vi "Filter Targets.vi"(6 "Camera Type":enum16{"206", "1011"}(ring), 9 "Targets":T2[](array[typedef]), 10 "Score Limits":T3, 11 "Image Size":cluster{i32, i32}) -> (3 "Filtered Targets":T1[](array[typedef]))   [LabVIEW 2011]
uses:
  Target Data.ctl
  Target.ctl
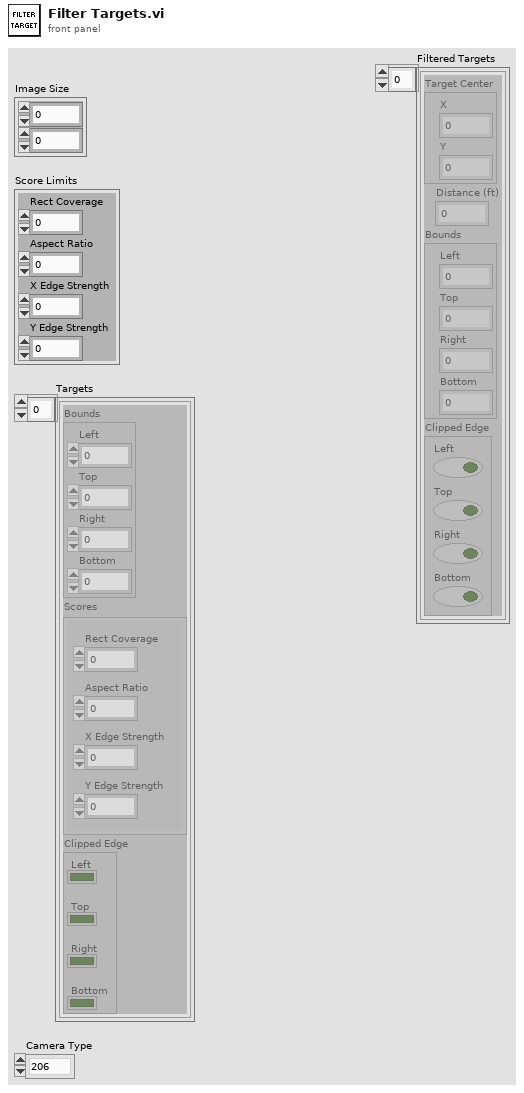
[diagram p1: front panel]
types:
  T1 = typedef "Target.ctl" = cluster{"Target Center":cluster{"X":dbl, "Y":dbl}, "Distance (ft)":dbl, "Bounds":cluster{"Left":dbl, "Top":dbl, "Right":dbl, "Bottom":dbl}, "Clipped Edge":cluster{"Left":bool, "Top":bool, "Right":bool, "Bottom":bool}}
  T2 = typedef "Target Data.ctl" = cluster{"Bounds":cluster{"Left":dbl, "Top":dbl, "Right":dbl, "Bottom":dbl}, "Scores":cluster{"Rect Coverage":dbl, "Aspect Ratio":dbl, "X Edge Strength":dbl, "Y Edge Strength":dbl}, "Clipped Edge":cluster{"Left":bool, "Top":bool, "Right":bool, "Bottom":bool}}
  T3 = cluster{"Rect Coverage":dbl, "Aspect Ratio":dbl, "X Edge Strength":dbl, "Y Edge Strength":dbl}
  T4 = cluster{"Left":dbl, "Top":dbl, "Right":dbl, "Bottom":dbl}
  T5 = cluster{"Left":bool, "Top":bool, "Right":bool, "Bottom":bool}
  T6 = cluster{"Target Center":cluster{"X":dbl, "Y":dbl}, "Distance (ft)":dbl, "Bounds":cluster{"Left":dbl, "Top":dbl, "Right":dbl, "Bottom":dbl}, "Clipped Edge":cluster{"Left":bool, "Top":bool, "Right":bool, "Bottom":bool}}
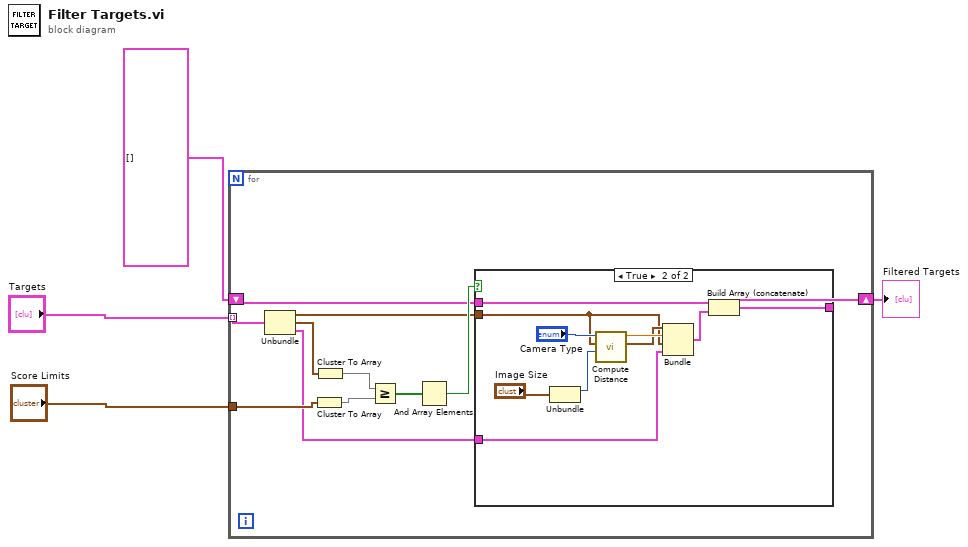
[diagram p0: block diagram]
diagram:
  n1 = for {
    tunnel: "Targets" -> [w15] mode=indexing
    tunnel: "Score Limits" -> [w13]
    shift-right: [w7] -> w1
    shift-left: T1[] [] -> [w8]
    n2 = Unbundle(w15) -> ("Bounds"=w6:T4, "Scores"=w14:T3, "Clipped Edge"=w5:T5)
    n3 = Cluster To Array(cluster=w13) -> (array=w11:dbl[])
    n4 = Cluster To Array(cluster=w14) -> (array=w12:dbl[])
    n5 = Greater Or Equal?(x=w12, y=w11) -> (x >= y?=w10:bool[])
    n6 = And Array Elements(Boolean array=w10) -> (logical AND=w9:bool)
    n7 = case shown="True" w9 {
      tunnel: w8 -> [w16 w26]
      tunnel: [w16 w25] -> w7
      tunnel: w6 -> [_ w18]
      tunnel: w5 -> [_ w17]
      frame False {
      }
      frame True {
        n8 = Unbundle("Image Size") -> (w19:i32)  [unwired: 1 out]
        n9 = call "Compute Distance.vi"("X Image Resolution"=w19, "Bounding Box"=w18, "Camera Type"="Camera Type") -> ("Target Center"=w22:cluster{"X":dbl, "Y":dbl}, "Distance (ft)"=w23:dbl)  [unwired: 7 in]
        n10 = Bundle("Target Center"=w22, "Distance (ft)"=w23, "Bounds"=w18, "Clipped Edge"=w17) -> (w24:T6)  [unwired: 1 in]
        n11 = Build Array (concatenate)(w26, w24) -> (w25:T1[])
      }
    }
  }
  "Filtered Targets" <- w1
